vi "Test Find Shortest.vi"(11 "Test Case In":refnum<class "Numeric Keypad Test.lvclass">) -> (0 "error out":errorcluster, 3 "Test Case Out":refnum<class "Numeric Keypad Test.lvclass">)   [LabVIEW 2020, in "Numeric Keypad Test.lvclass"]
uses:
  Numeric Keypad Test.lvclass
  C:/Program Files (x86)/National Instruments/LabVIEW 2020/vi.lib/Astemes/LUnit/Test Case.lvclass
  Numeric Keypad Test.lvclass/Numeric Keypad Test.ctl
  <vilib>/Astemes/LUnit/Test Case.lvclass/Test Case.ctl
  <vilib>/Astemes/LUnit/Append Pass Result.vi
  <vilib>/Astemes/LUnit/Append Fail Result.vi
  <vilib>/Astemes/LUnit/Describe Comparison.vi
  4993e8ee-a06a-463a-9684-69129f64d5ce.vi/9c5d11cd-9439-4240-a1ee-d9baace9c924.vi
  <vilib>/Astemes/LUnit/Run In UI.vi
  <vilib>/Utility/error.llb/Clear Errors.vi
  <vilib>/Astemes/LUnit/Describe Variant.vi
  Numeric Keypad/Numeric Keypad.lvclass
  46ac11b3-c1d7-4248-9e11-9ad0b7b42e7d.vi
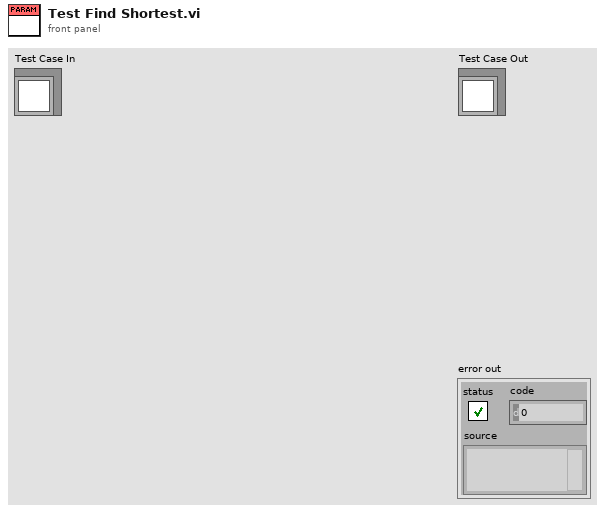
[diagram p1: front panel]
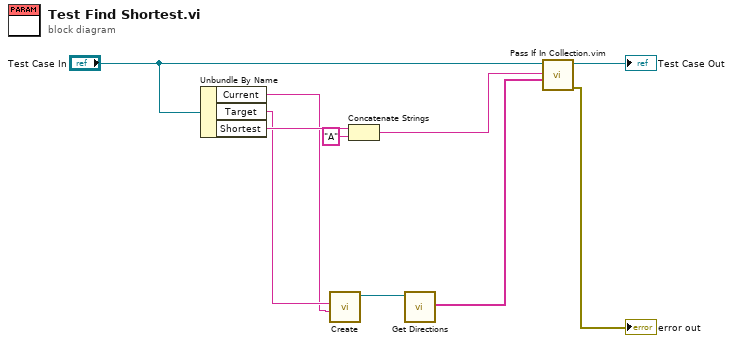
[diagram p0: block diagram]
diagram:
  n1 = Unbundle By Name("Test Case In") -> ("Current"=w3:string, "Target"=w4:string, "Shortest"=w6:string)
  n2 = call "Create.vi"("Current"=w3, "Input"=w4) -> ("Proto"=w7:refnum<class "Numeric Keypad.lvclass">)  [unwired: 9 in]
  n3 = Concatenate Strings(w6, "A" ("string")) -> (w2:string)
  n4 = call "Get Directions.vi"("Proto in"=w7) -> ("Directional Button Presses"=w5:string[])  [unwired: 9 in, 1 out]
  n5 = call "Pass If In Collection.vim"("Collection"=w5, "Expected Element"=w2, "LUnit Test Case In"="Test Case In") -> ("error out"=→"error out":errorcluster, "LUnit Test Case Out"=→"Test Case Out":refnum<class "Numeric Keypad Test.lvclass">)  [unwired: 7 in]
